vi "readAvailable.vi"(8 "error in (no error)":errorcluster, 11 "SerialProtocol in":refnum<class "SerialProtocol.lvclass">) -> (0 "error out":errorcluster, 2 "stringRead":string, 3 "SerialProtocol out":refnum<class "SerialProtocol.lvclass">)   [LabVIEW 2015, in "SerialProtocols.lvlib" / "SerialProtocol.lvclass"]
uses:
  <userlib>/Common/SerialProtocols/SerialProtocol/SerialProtocol/SerialProtocol.lvclass
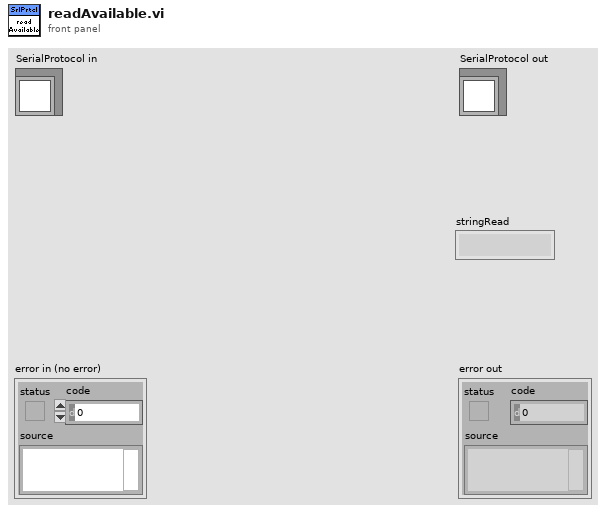
[diagram p1: front panel]
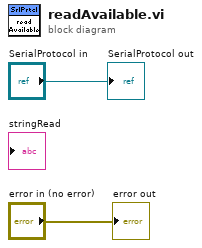
[diagram p0: block diagram]
diagram:
  "error out" <- "error in (no error)"
  "SerialProtocol out" <- "SerialProtocol in"
